vi "Práctica01_Ejercicio2_3.vi"() -> ()   [LabVIEW 2020]
panel:
  out "Thermometer":dbl(slide) scale=25.0..100.0
  out "Tank":dbl(slide) scale=0.0..20.0
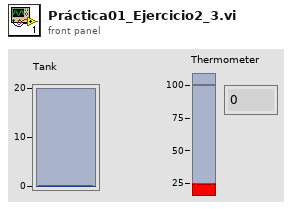
[diagram p1: front panel]
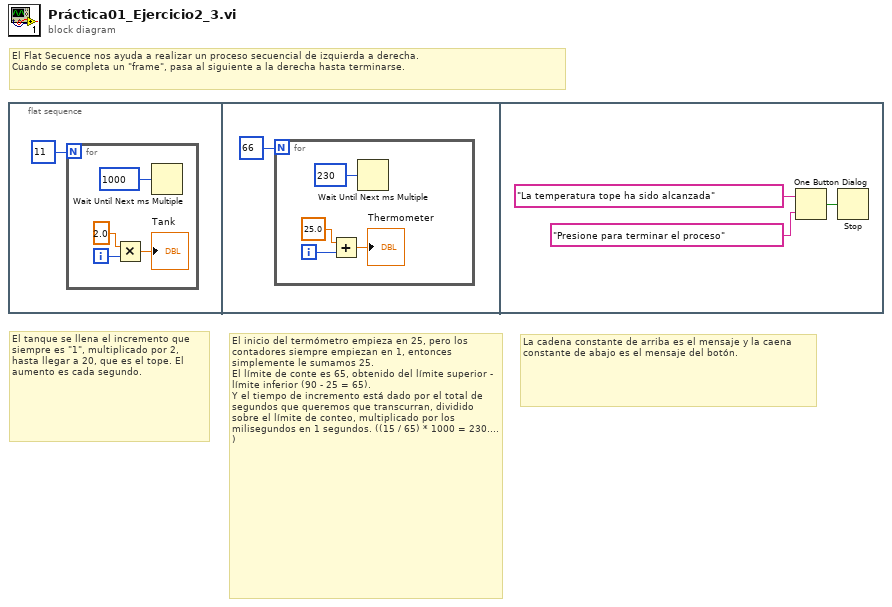
[diagram p0: block diagram]
diagram:
  # "El Flat Secuence nos ayuda a realizar un proceso secuencial de izquierda a derecha.\nCuando se completa un \"frame\", pasa al siguiente a la derecha hasta terminarse."
  # "La cadena constante de arriba es el mensaje y la caena constante de abajo es el mensaje del botón."
  # "El inicio del termómetro empieza en 25, pero los contadores siempre empiezan en 1, entonces simplemente le sumamos 25. \nEl límite de conte es 65, obtenido del límite superior - límite inferior (90 - 25 = 65).\nY el tiempo de incremento está dado por el total de segundos que queremos que transcurran, dividido sobre el límite de conteo, multiplicado por los milisegundos en 1 segundos. ((15 / 65) * 1000 = 230....)"
  # "El tanque se llena el incremento que siempre es \"1\", multiplicado por 2, hasta llegar a 20, que es el tope. El aumento es cada segundo."
  n1 = flat-sequence {
    frame #0 {
      n2 = for {
        N: 11 -> [_]
        i -> [w4]
        n3 = Multiply(x=2.0, y=w4) -> (x*y=→"Tank":dbl)
        n4 = Wait Until Next ms Multiple(millisecond multiple=u32 1000) -> ()  [unwired: 1 out]
      }
    }
    frame #1 {
      n5 = for {
        N: 66 -> [_]
        i -> [w9]
        n6 = Add(x=25.0, y=w9) -> (x+y=→"Thermometer":dbl)
        n7 = Wait Until Next ms Multiple(millisecond multiple=u32 230) -> ()  [unwired: 1 out]
      }
    }
    frame #2 {
      n8 = One Button Dialog(message="La temperatura tope ha sido alcanzada", button name ("OK")="Presione para terminar el proceso") -> (true=w11:bool)
      n9 = Stop(stop? (T)=w11) -> ()
    }
  }
